vi "reqwest_async_cleanup.vi"(8 "error in (no error)":errorcluster, 11 "Request in":refnum<class "Request.lvclass">) -> (0 "error out":errorcluster, 2 "success":bool)   [LabVIEW 2020, in "reqwest.lvlib" / "Request.lvclass"]
uses:
  Request.lvclass
  Request.lvclass/Request.ctl
  lv_reqwest_64.dll
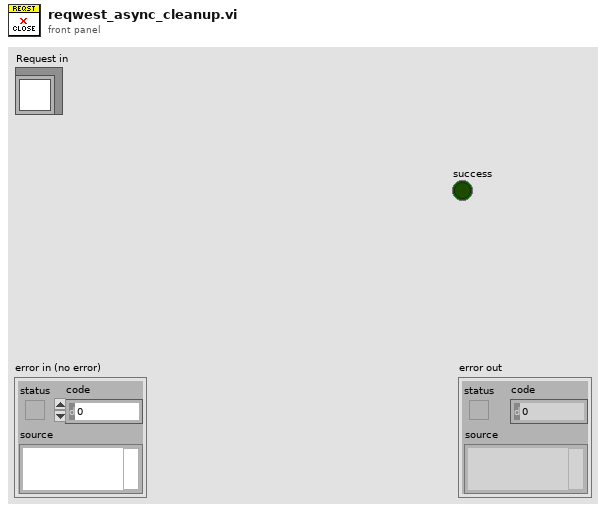
[diagram p1: front panel]
types:
  T1 = typedef "reqwest.lvlib/Request.lvclass/request_id_int.ctl" = i32
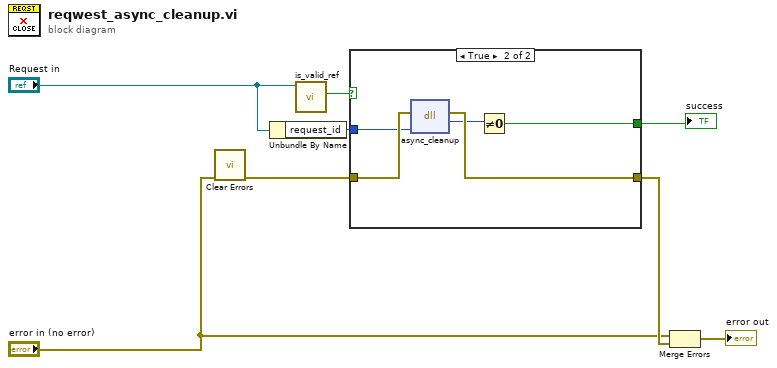
[diagram p0: block diagram]
diagram:
  n1 = call <vilib>:"Clear Errors.vi"("error in (no error)"="error in (no error)") -> ("error out"=w7:errorcluster)  [unwired: 5 in, 1 out]
  n2 = Unbundle By Name("Request in") -> ("request_id"=w4:T1)
  n3 = call "is_valid_ref.vi"("Request in"="Request in") -> ("valid-ref?"=w2:bool)  [unwired: 10 in]
  n4 = case shown="True" w2 {
    tunnel: [w9 w14] -> w8
    tunnel: w7 -> [w9 w13]
    tunnel: w4 -> [_ w12]
    tunnel: [_ w10] -> w1
    frame False {
    }
    frame True {
      n5 = dll-call lib="C:/Projects/reqwest-rs-labview/lv_src/lv_reqwest_64.dll" fn="async_cleanup"(error in=w13, "request_id"=w12) -> (error out=w14:errorcluster, "success"=w11:u8)  [unwired: 3 in, 1 out]
      n6 = Not Equal To 0?(x=w11) -> (x != 0?=w10:bool)
    }
  }
  "success" <- w1
  n7 = Merge Errors("error in (no error)", w8) -> (→"error out":errorcluster)
